vi "Initialize.vi"(8 "error in (no error)":errorcluster, 11 "RDMA Plugin User Interface in":refnum<class "RDMA Plugin User Interface.lvclass">) -> (0 "error out":errorcluster, 3 "RDMA Plugin User Interface out":refnum<class "RDMA Plugin User Interface.lvclass">)   [LabVIEW 2020, in "RDMA.lvlib" / "RDMA Plugin User Interface.lvclass"]
uses:
  RDMA Plugin User Interface.lvclass
  Configuration/Plugin/RDMA Plugin Configuration.lvclass
  DSF Core.lvlibp/Classes/User Interface/User Interface.lvclass
  C:/git/fmussi-niveristand-data-sharing-framework-custom-device-plugins/Components/DSF Core.lvlibp/Classes/Configuration/Configuration.lvclass
  C:/git/fmussi-niveristand-data-sharing-framework-custom-device-plugins/Components/DSF Core.lvlibp/Classes/User Interface/User Interface.lvclass
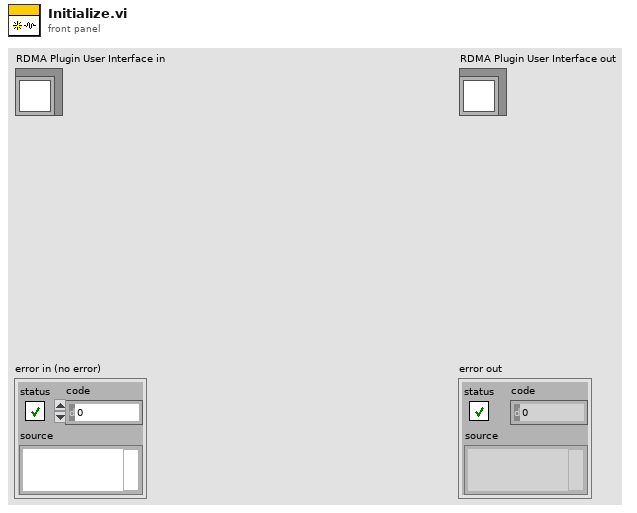
[diagram p1: front panel]
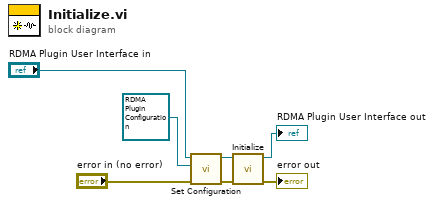
[diagram p0: block diagram]
diagram:
  n1 = call "Set Configuration.vi"("error in (no error)"="error in (no error)", "configuration"=refnum<class "RDMA Plugin Configuration.lvclass"> refnum ("RDMA.lvlib:RDMA Plugin Configuration.lvclass"), "User Interface in"="RDMA Plugin User Interface in") -> ("error out"=w3:errorcluster, "User Interface out"=w4:refnum<class "RDMA Plugin User Interface.lvclass">)  [unwired: 7 in]
  n2 = call-parent "Initialize.vi"("error in (no error)"=w3, "User Interface in"=w4) -> ("error out"=→"error out":errorcluster, "User Interface out"=→"RDMA Plugin User Interface out":refnum<class "RDMA Plugin User Interface.lvclass">)  [unwired: 8 in]
